vi "Start.vi"(8 "Error In":errorcluster, 11 "object in":refnum<class "IGenerate Waveform.lvclass">) -> (0 "Error Out":errorcluster, 3 "object out":refnum<class "IGenerate Waveform.lvclass">)   [LabVIEW 2023, in "HAL Interfaces.lvlib" / "IGenerate Waveform.lvclass"]
uses:
  IGenerate Waveform.lvclass
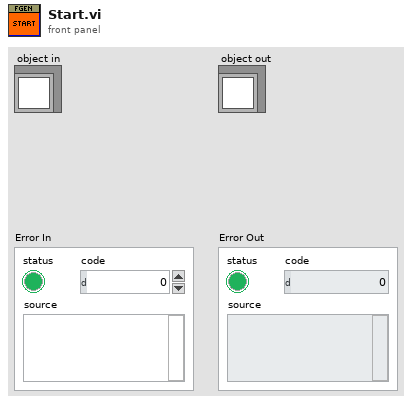
[diagram p1: front panel]
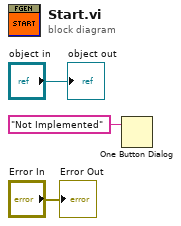
[diagram p0: block diagram]
diagram:
  n1 = One Button Dialog(message="Not Implemented") -> ()  [unwired: 1 in, 1 out]
  "Error Out" <- "Error In"
  "object out" <- "object in"
